vi "校准数据选择表.vi"(9 "测量模式":T1(ring), 10 "量程下拉列表":enum16{"低量程", "高量程"}(ring), 11 "table":string="氨氮") -> (2 "布尔":bool=TRUE, 3 "输出":T2)   [LabVIEW 2016, in "斯坦道总磷总氮V2.lvlib"]
uses:
  <vilib>/Utility/miscctls.llb/LVPointTypeDef.ctl
  <vilib>/Utility/miscctls.llb/LVRowAndColumnUnsignedTypeDef.ctl
panel:
  in  "吸光值选择：":enum16{"X", "F2"}(ring)
  in  "显示全部数据":bool caption="显示全部数据："
  in  "确定":bool
  in  "返回":bool
  in  "多列列表框":i32(listbox)
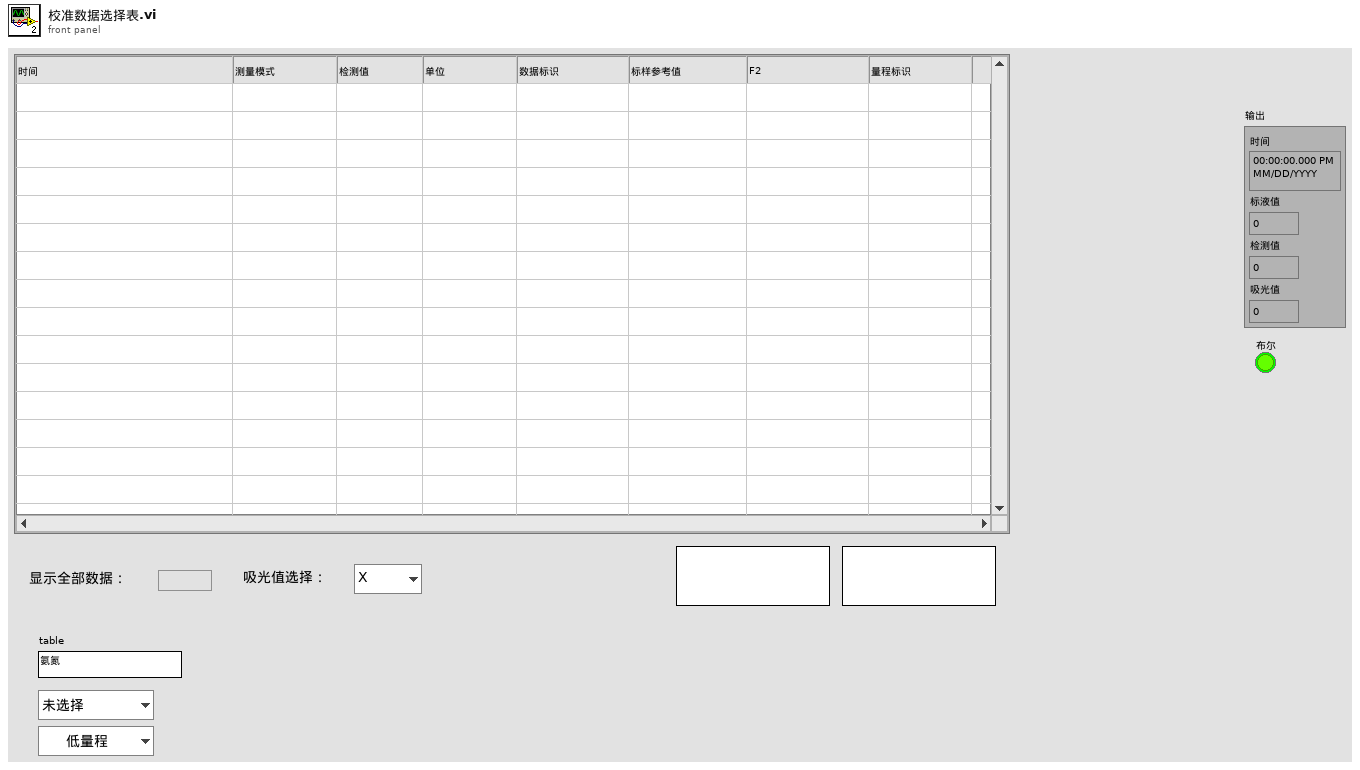
[diagram p1: front panel]
types:
  T1 = enum16{"未选择", "空白校准", "标样校准", "标样核查", "零点核查", "跨度核查"}
  T2 = cluster{"时间":timestamp, "标液值":dbl, "检测值":dbl, "吸光值":dbl}
  T3 = typedef "LVRowAndColumnUnsignedTypeDef.ctl" = cluster{"Row":u32, "Column":u32}
  T4 = typedef "LVPointTypeDef.ctl" = cluster{"Horizontal":i16, "Vertical":i16}
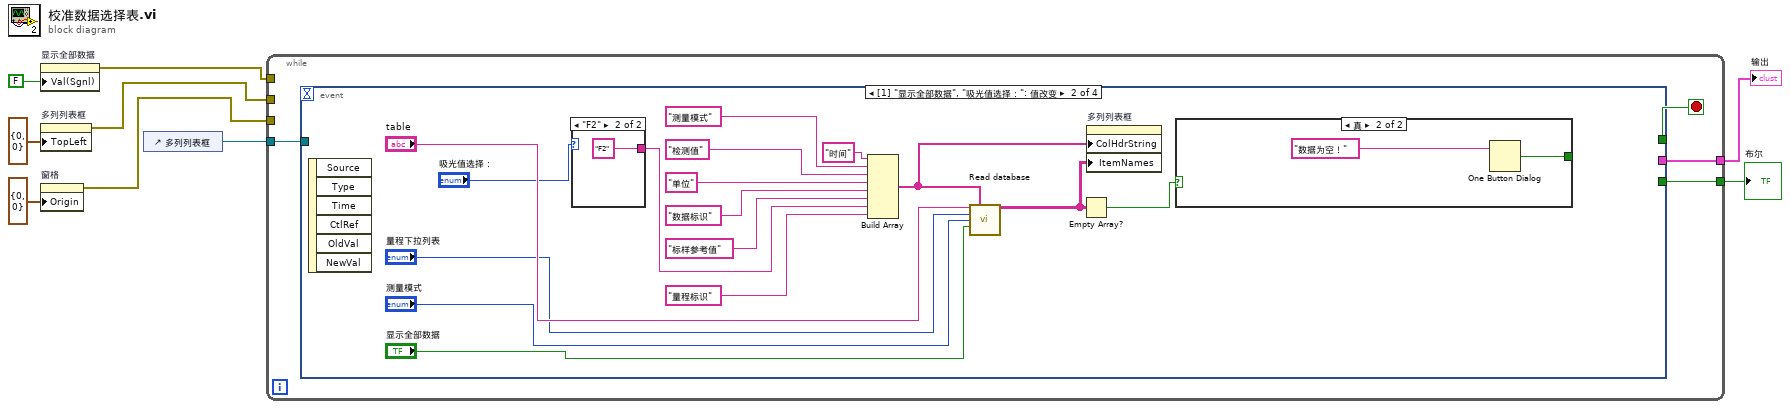
[diagram p0: block diagram]
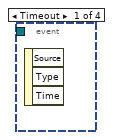
[diagram p2: hidden frame]
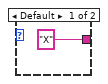
[diagram p3: hidden frame]
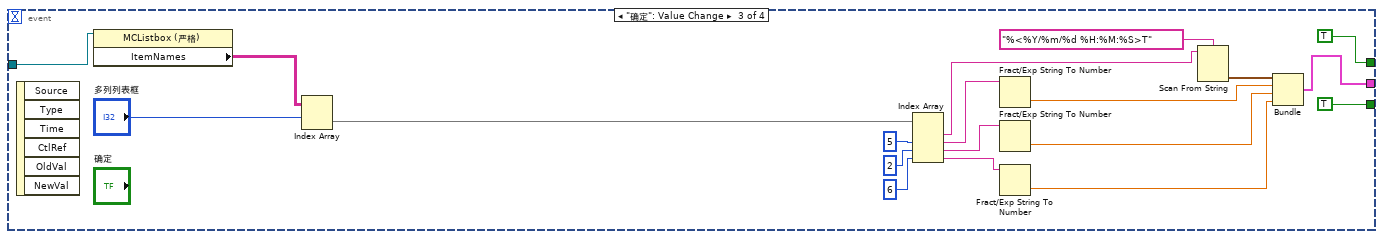
[diagram p5: hidden frame]
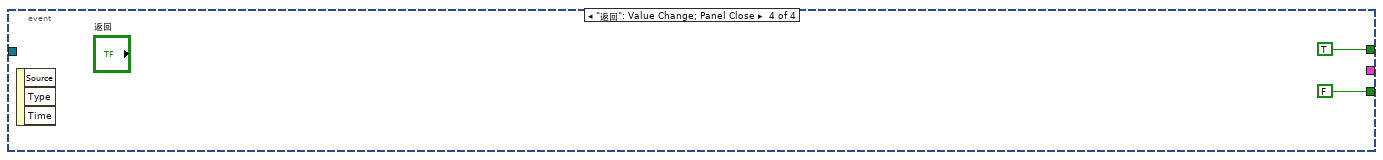
[diagram p6: hidden frame]
diagram:
  n1 = property on="显示全部数据" class="Bool (严格)"("Val(Sgnl)"=FALSE ("值(信号)")) -> (error out=w2:errorcluster)  [unwired: 2 in, 1 out]
  n2 = property on="多列列表框" class="MCListbox (严格)"("TopLeft"=T3 {"Row"=0, "Column"=0} ("左上可见单元格")) -> (error out=w3:errorcluster)  [unwired: 2 in, 1 out]
  n3 = property on="窗格" class="Pane"("Origin"=T4 {"Horizontal"=0, "Vertical"=0} ("原点")) -> (error out=w8:errorcluster)  [unwired: 2 in, 1 out]
  n4 = control-ref of="多列列表框"() -> (w5:refnum<vi>)
  n5 = while {
    tunnel: w5 -> [w12]
    tunnel: w8 -> [_]
    tunnel: [w11] -> w7
    tunnel: [w10] -> w6
    tunnel: w3 -> [_]
    tunnel: w2 -> [_]
    stop <- w13 stop-if-true
    n6 = event shown="[1] \"显示全部数据\", \"吸光值选择：\": 值改变" {
      selector: _ -> [_ _ _ _]
      dyn-events: _ -> [_ _ _ _]
      timeout: _ -> [_ _ _ _]
      tunnel: [_ _ TRUE TRUE] -> w13
      tunnel: w12 -> [_ _ w50 _]
      tunnel: [_ _ TRUE FALSE] -> w11
      tunnel: [_ _ w37 _] -> w10
      event Timeout {
        n7 = event-data() -> ()  [unwired: 1 in, 3 out]
      }
      event "显示全部数据", "吸光值选择：": Value Change {
        n8 = event-data() -> ()  [unwired: 1 in, 6 out]
        n9 = case shown="\"F2\"" "吸光值选择：" {
          tunnel: ["X" "F2"] -> w27
          frame Default {
          }
          frame "F2" {
          }
        }
        n10 = Build Array("时间", "测量模式", "检测值", "单位", "数据标识", "标样参考值", w27, "量程标识") -> (w23:string[])
        n11 = call "Read database.vi"("table"="table", "显示项"=w23, "量程下拉列表"="量程下拉列表", "测量模式"="测量模式", "显示全部数据"="显示全部数据") -> ("表格"=w15:string[][])  [unwired: 7 in, 3 out]
        n12 = Empty Array?(array=w15) -> (empty?=w16:bool)
        n13 = property on="多列列表框" class="MCListbox (严格)"("ColHdrString"=w23, "ItemNames"=w15) -> ()  [unwired: 2 in, 2 out]
        n14 = case shown="真" w16 {
          tunnel: [_ w32] -> _
          frame False {
          }
          frame True {
            n15 = One Button Dialog(message="数据为空！" ("消息")) -> (true=w32:bool)  [unwired: 1 in]
          }
        }
      }
      event "确定": Value Change {
        n16 = event-data() -> ()  [unwired: 1 in, 6 out]
        n17 = property class="MCListbox (严格)"(reference=w50) -> ("ItemNames"=w51:string[][])  [unwired: 1 in, 2 out]
        n18 = Index Array(array=w51, index (row)="多列列表框") -> (element=w47:string[])  [unwired: 1 in]
        n19 = Index Array(array=w47, index #2=5 ("索引"), index #3=2 ("索引"), index #4=6 ("索引")) -> (element #1=w35:string, element #2=w43:string, element #3=w42:string, element #4=w41:string)  [unwired: 1 in]
        n20 = Fract/Exp String To Number(string=w43) -> (number=w40:dbl)  [unwired: 3 in, 1 out]
        n21 = Fract/Exp String To Number(string=w42) -> (number=w39:dbl)  [unwired: 3 in, 1 out]
        n22 = Fract/Exp String To Number(string=w41) -> (number=w38:dbl)  [unwired: 3 in, 1 out]
        n23 = Scan From String(format string="%<%Y/%m/%d %H:%M:%S>T" ("格式字符串"), input string=w35) -> (output 1=w34:timestamp)  [unwired: 3 in, 3 out]
        n24 = Bundle(w34, w40, w39, w38) -> (w37:cluster{timestamp, dbl, dbl, dbl})  [unwired: 1 in]
      }
      event "返回": Value Change; Panel Close {
        n25 = event-data() -> ()  [unwired: 1 in, 3 out]
      }
    }
  }
  "布尔" <- w7
  "输出" <- w6
